vi "New Config.vi"(8 "error in (no error)":errorcluster, 10 "New Config":T1, 11 "System Config Module in":refnum<class "System Config Module.lvclass">) -> (0 "error out":errorcluster, 3 "System Config Module out":refnum<class "System Config Module.lvclass">)   [LabVIEW 2020, in "Volatus.lvlib" / "System Config Module.lvclass"]
uses:
  System Config Module.lvclass
  C:/dev/lv20CE/relink/lv-volatus/Volatus/Module/Module.lvclass
  New Config.ctl
  Module/Module.lvclass/Module.ctl
  MessageQ/MessageQ.lvclass/MessageQ.ctl
  MessageQ/Send.vi
  Module/Parent Q.vi
  System Config Module.lvclass/System Config Module.ctl
  Module/Module.lvclass
  Volatus.lvlib
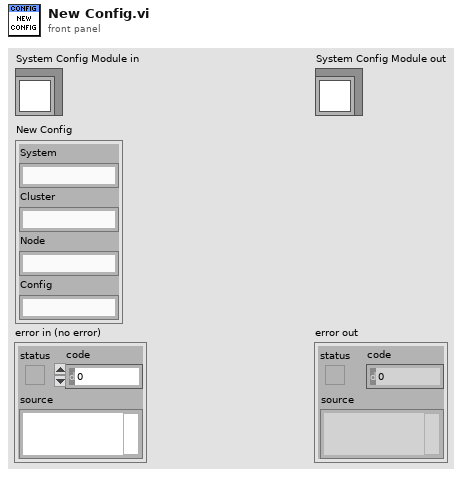
[diagram p1: front panel]
types:
  T1 = typedef "Volatus.lvlib/New Config.ctl" = cluster{"System":string, "Cluster":string, "Node":string, "Config":string}
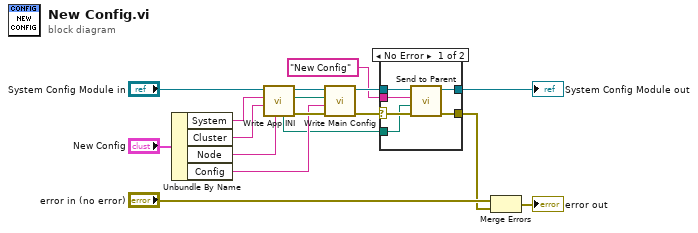
[diagram p0: block diagram]
diagram:
  n1 = Unbundle By Name("New Config") -> ("System"=w12:string, "Cluster"=w11:string, "Node"=w10:string, "Config"=w8:string)
  n2 = call "Write App INI.vi"("Node"=w10, "Cluster"=w11, "System"=w12, "System Config Module in"="System Config Module in") -> ("error out"=w17:errorcluster, "Main Config Path"=w7:path, "System Config Module out"=w13:refnum<class "System Config Module.lvclass">, "INI Path"=w1:path)  [unwired: 4 in]
  n3 = call "Write Main Config.vi"("error in (no error)"=w17, "Config"=w8, "Main Config Path"=w7, "System Config Module in"=w13) -> ("error out"=w4:errorcluster, "System Config Module out"=w9:refnum<class "System Config Module.lvclass">)  [unwired: 6 in]
  n4 = case shown="No Error" w4 {
    selector: w4 -> [w21 w24]
    tunnel: w9 -> [w23 w25]
    tunnel: [w22 w25] -> w5
    tunnel: "New Config" ("Message ID") -> [w20 _]
    tunnel: [w19 w24] -> w2
    tunnel: w1 -> [w18 _]
    frame No Error {
      n5 = call "Send to Parent.vi"("error in (no error)"=w21, "Data"=w18, "Message ID"=w20, "Module in"=w23) -> ("error out"=w19:errorcluster, "Module out"=w22:refnum<class "System Config Module.lvclass">)  [unwired: 6 in]
    }
    frame Error {
    }
  }
  "System Config Module out" <- w5
  n6 = Merge Errors("error in (no error)", w2) -> (→"error out":errorcluster)
